vi "Open Existing Track.vi"(8 "error in (no error)":errorcluster, 11 "Track Name":string) -> (0 "error out":errorcluster, 3 "Track (File) References":T1)   [LabVIEW 2014]
doc: "Open an existing Audio File and Return the File reference."
uses:
  Controls/Track (File) References.ctl
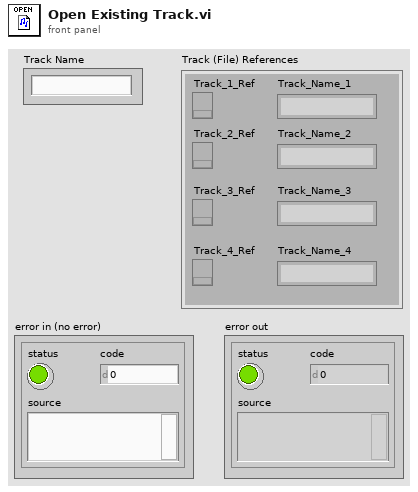
[diagram p1: front panel]
types:
  T1 = typedef "Track (File) References.ctl" = cluster{"Track_1_Ref":refnum<k34>, "Track_2_Ref":refnum<k34>, "Track_3_Ref":refnum<k34>, "Track_4_Ref":refnum<k34>, "Track_Name_1":string, "Track_Name_2":string, "Track_Name_3":string, "Track_Name_4":string}
  T2 = typedef "Track File Names.ctl" = cluster{"Track_1":string, "Track_2":string, "Track_3":string, "Track_4":string}
  T3 = cluster{"Track_1_Path":path, "Track_2_Path":path, "Track_3_Path":path, "Track_4_Path":path}
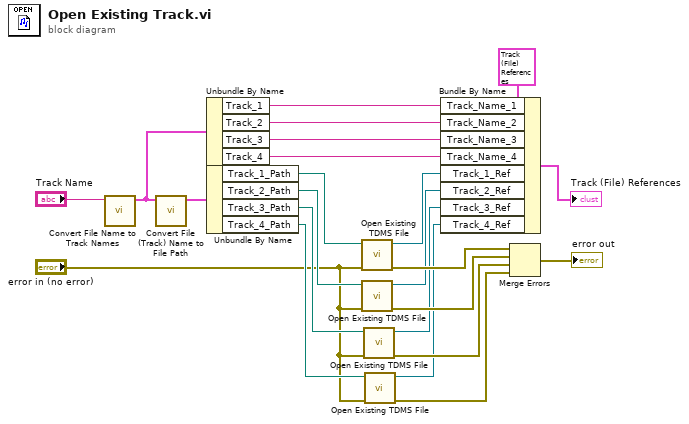
[diagram p0: block diagram]
diagram:
  n1 = call "Convert File Name to Track Names.vi"("File Name"="Track Name") -> ("Track Names"=w5:T2)  [unwired: 10 in]
  n2 = call "Convert File (Track) Name to File Path.vi"("Track Names"=w5) -> ("Track File Paths"=w22:T3)  [unwired: 10 in]
  n3 = Unbundle By Name(w5) -> ("Track_1"=w4:string, "Track_2"=w3:string, "Track_3"=w2:string, "Track_4"=w1:string)
  n4 = Unbundle By Name(w22) -> ("Track_1_Path"=w21:path, "Track_2_Path"=w20:path, "Track_3_Path"=w19:path, "Track_4_Path"=w18:path)
  n5 = call "Open Existing TDMS File.vi"("Error In"="error in (no error)", "TDMS File Path"=w21) -> ("Error Out"=w16:errorcluster, "TDMS File Ref Out"=w9:refnum<k34>)  [unwired: 8 in]
  n6 = call "Open Existing TDMS File.vi"("Error In"="error in (no error)", "TDMS File Path"=w20) -> ("Error Out"=w15:errorcluster, "TDMS File Ref Out"=w8:refnum<k34>)  [unwired: 8 in]
  n7 = call "Open Existing TDMS File.vi"("Error In"="error in (no error)", "TDMS File Path"=w19) -> ("Error Out"=w14:errorcluster, "TDMS File Ref Out"=w7:refnum<k34>)  [unwired: 8 in]
  n8 = call "Open Existing TDMS File.vi"("Error In"="error in (no error)", "TDMS File Path"=w18) -> ("Error Out"=w13:errorcluster, "TDMS File Ref Out"=w6:refnum<k34>)  [unwired: 8 in]
  n9 = Bundle By Name(cluster=T1 {"Track_1_Ref"=refnum, "Track_2_Ref"=refnum, "Track_3_Ref"=refnum, "Track_4_Ref"=refnum, "Track_Name_1"="", "Track_Name_2"="", "Track_Name_3"="", "Track_Name_4"=""} ("Track (File) References"), "Track_Name_1"=w4, "Track_Name_2"=w3, "Track_Name_3"=w2, "Track_Name_4"=w1, "Track_1_Ref"=w9, "Track_2_Ref"=w8, "Track_3_Ref"=w7, "Track_4_Ref"=w6) -> (→"Track (File) References":T1)
  n10 = Merge Errors(w16, w15, w14, w13) -> (→"error out":errorcluster)
